vi "ConvertToVoltsArray.vi"(10 "Voltage Range":dbl=10.0 format="%#_13g", 11 "Channels":i16[](array[numeric])) -> (2 "Volts":dbl[](array[numeric]))   [LabVIEW 2016]
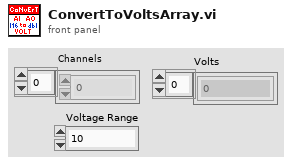
[diagram p1: front panel]
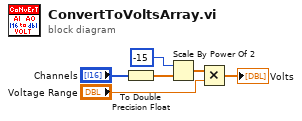
[diagram p0: block diagram]
diagram:
  n1 = To Double Precision Float(number="Channels") -> (double precision float=w3:dbl[])
  n2 = Scale By Power Of 2(n=i16 -15, x=w3) -> (x*2^n=w5:dbl[])
  n3 = Multiply(x=w5, y="Voltage Range") -> (x*y=→"Volts":dbl[])
